vi "PID COPPIA.vi"(0 "setpoint":dbl format="%.2f", 1 "Max":dbl, 2 "%max":dbl format="%#_13g", 3 "output low pid =0":bool, 5 "process variable":dbl format="%.2f", 7 "PID gains":T1={"proportional gain (Kc)"=0.4, "integral time (Ti, min)"=0.025, "derivative time (Td, min)"=0.0} {"derivative time (Td, min)" format="%.3f"; "integral time (Ti, min)" format="%.3f"; "proportional gain (Kc)" format="%.3f"}, 8 "Pid in pausa":bool, 9 "sample length":i32=10, 11 "dt (s)":dbl=-1.0 format="%.3f", 12 "Precisione":dbl=0.015 format="%#_13g", 13 "Abilita pid":bool=TRUE, 14 "initialize pid":bool, 15 "Escludi init new value":bool) -> (4 "output":dbl, 10 "Stabile?":bool)   [LabVIEW 2019]
uses:
  <vilib>/addons/control/pid/pid.llb/PID (DBL).vi
  <vilib>/addons/control/pid/NI_PID_pid.lvlib
  <vilib>/ptbypt/NI_PtbyPt.lvlib
panel:
  in  "initialize":bool
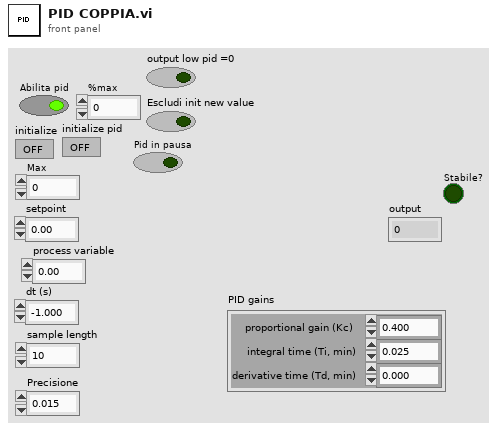
[diagram p1: front panel]
types:
  T1 = cluster{"proportional gain (Kc)":dbl, "integral time (Ti, min)":dbl, "derivative time (Td, min)":dbl}
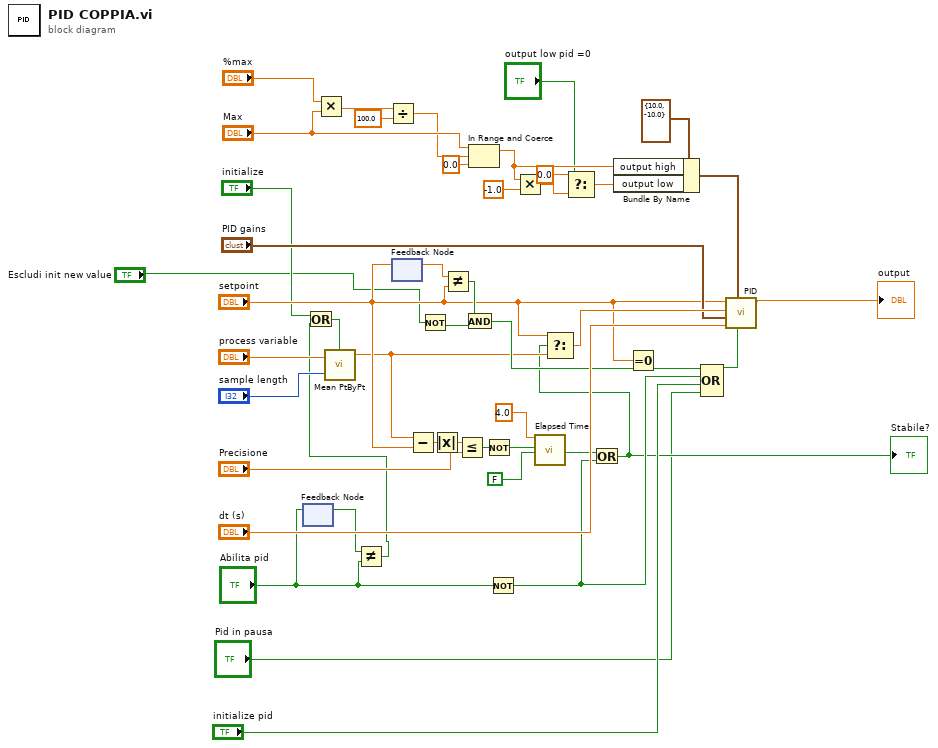
[diagram p0: block diagram]
diagram:
  n1 = feedback-in #1("Abilita pid") -> ()
  n2 = feedback #1() -> (w14:bool)  [unwired: 1 in]
  n3 = Multiply(x="%max", y="Max") -> (x*y=w25:dbl)
  n4 = Not Equal?(x=w14, y="Abilita pid") -> (x != y?=w12:bool)
  n5 = Or(x="initialize", y=w12) -> (x .or. y?=w15:bool)
  n6 = call <vilib>:"Mean PtByPt.vi"("x"="process variable", "sample length"="sample length", "initialize"=w15) -> ("mean"=w4:dbl)  [unwired: 1 in, 1 out]
  n7 = Divide(x=w25, y=100.0) -> (x/y=w18:dbl)
  n8 = feedback-in #2("setpoint") -> ()
  n9 = feedback #2() -> (w36:dbl)  [unwired: 1 in]
  n10 = Subtract(x=w4, y="setpoint") -> (x-y=w42:dbl)
  n11 = Not(x="Escludi init new value") -> (.not. x?=w6:bool)
  n12 = Absolute Value(x=w42) -> (abs(x)=w40:dbl)
  n13 = Not Equal?(x=w36, y="setpoint") -> (x != y?=w34:bool)
  n14 = Less Or Equal?(x=w40, y="Precisione") -> (x <= y?=w29:bool)
  n15 = And(x=w34, y=w6) -> (x .and. y?=w7:bool)
  n16 = In Range and Coerce(upper limit="Max", x=w18, lower limit=0.0) -> (coerced(x)=w19:dbl)  [unwired: 1 out]
  n17 = Not(x=w29) -> (.not. x?=w30:bool)
  n18 = Not(x="Abilita pid") -> (.not. x?=w27:bool)
  n19 = Multiply(x=w19, y=-1.0) -> (x*y=w11:dbl)
  n20 = call "Elapsed Time"("Time Target (s)"=4.0, "Reset"=w30, "Auto Reset"=FALSE) -> ("Time has Elapsed"=w3:bool)  [unwired: 9 in, 7 out]
  n21 = Select(t=0.0, s="output low pid =0", f=w11) -> (s? t:f=w10:dbl)
  n22 = Or(x=w3, y=w27) -> (x .or. y?=w2:bool)
  "Stabile?" <- w2
  n23 = Select(t="setpoint", s=w2, f=w4) -> (s? t:f=w41:dbl)
  n24 = Bundle By Name(cluster=cluster{"output high":dbl, "output low":dbl} {"output high"=10.0, "output low"=-10.0} ("output range"), "output high"=w19, "output low"=w10) -> (w38:cluster{"output high":dbl, "output low":dbl})
  n25 = Equal To 0?(x="setpoint") -> ()  [unwired: 1 out]
  n26 = Compound Arithmetic op=OR(w7, w27, "initialize pid", "Pid in pausa") -> (w35:bool)
  n27 = call-poly <vilib>:"PID.vi"("reinitialize? (F)"=w35, "output range"=w38, "dt (s)"="dt (s)", "PID gains"="PID gains", "process variable"=w41, "setpoint"="setpoint") -> ("output"=→"output":dbl)  [unwired: 4 in, 1 out]
